vi "LoopScript_ChangeTime.vi"() -> ()   [LabVIEW 2017]
uses:
  FrontPanelReferences.vi
  Desktop/AODExperimentControls/ImageAcquisitionProgram/ImageAcquisitionLibrary/GlobalFrontPanelReferences.vi
  Desktop/AODExperimentControls/AODControl/AODGlobals.vi
  Desktop/AODExperimentControls/AODControl/MessageQueue/QueueOperations/Enqueue Message (Single).vi
  Desktop/AODExperimentControls/ImageAcquisitionProgram/ImageAcquisitionLibrary/ImageAcquisitionLibrary.lvlib
  Desktop/AODExperimentControls/AODControl/AODControl.lvlib
  Desktop/AODExperimentControls/AODControl/MessageQueue/MessageQueue.lvlib
panel:
  out "Current Radius":dbl
  in  "R_f":dbl
  in  "R_0":dbl
  in  "Radius Steps":i32=30
  out "Current Step Down":i32
  out "Current Step Up":i32
  out "Current Loop":i32
  in  "NumberOfLoops":i32
  in  "Record Time":u32=15000
  in  "B_f^2":dbl
  in  "B_0^2":dbl
  in  "Steps":i32=30
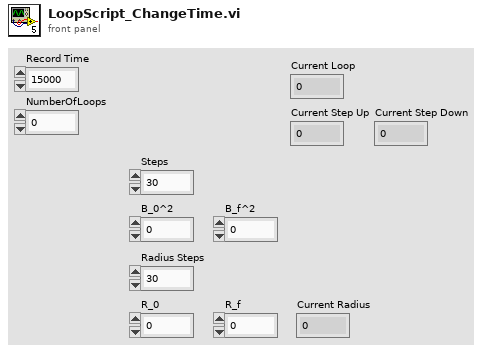
[diagram p1: front panel]
types:
  T1 = typedef "AODControl.lvlib/MessageQueue.lvlib/All Message Queues.ctl" = cluster{" AOD Interface":refnum<queue>}
  T2 = typedef "ImageAcquisitionLibrary.lvlib/References.ctl" = cluster{"Acquire":refnum<vi>, "Rec":refnum<vi>, "Tracking":refnum<vi>, "Settings":refnum<vi>, "Stop":refnum<vi>, "Initialized?":bool, "ImDisplay":refnum<vi>}
  T3 = typedef "WaveformGenerator.lvlib/WaveformGeneratorInterfaceRef.ctl" = cluster{"Waveform X":refnum<vi>, "Waveform Y":refnum<vi>, "Waveform Z":refnum<vi>, "Amplitude X":refnum<vi>, "Amplitude Y":refnum<vi>, "Amplitude Z":refnum<vi>, "Frequency X":refnum<vi>, "Frequency Y":refnum<vi>, "Frequency Z":refnum<vi>, "Phase X":refnum<vi>, "Phase Y":refnum<vi>, "Phase Z":refnum<vi>, "Offset X":refnum<vi>, "Offset Y":refnum<vi>, "Offset Z":refnum<vi>, "Stop":refnum<vi>, "On/Off":refnum<vi>, "Field^2":refnum<vi>}
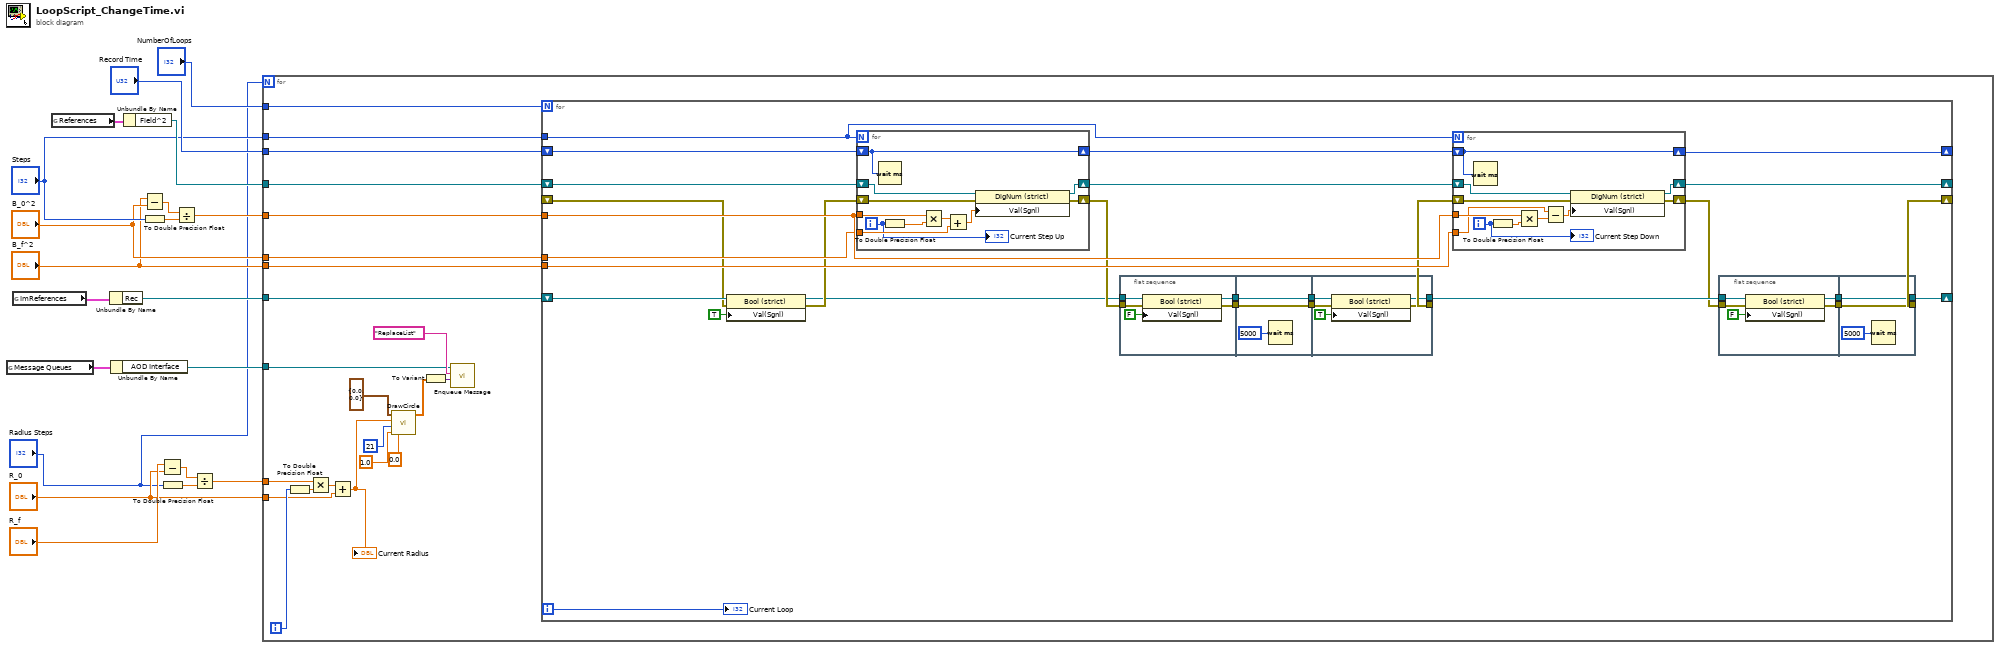
[diagram p0: block diagram]
diagram:
  n1 = global read "AODGlobals.vi" "Message Queues"() -> (w8:T1)
  n2 = global read "GlobalFrontPanelReferences.vi" "ImReferences"() -> (w10:T2)
  n3 = global read "FrontPanelReferences.vi" "References"() -> (w20:T3)
  n4 = Unbundle By Name(w10) -> ("Rec"=w9:refnum<vi>)
  n5 = Unbundle By Name(w8) -> ("AOD Interface"=w7:refnum<queue>)
  n6 = Unbundle By Name(w20) -> ("Field^2"=w19:refnum<vi>)
  n7 = Subtract(x="B_f^2", y="B_0^2") -> (x-y=w17:dbl)
  n8 = To Double Precision Float(number="Steps") -> (double precision float=w18:dbl)
  n9 = Subtract(x="R_f", y="R_0") -> (x-y=w6:dbl)
  n10 = To Double Precision Float(number="Radius Steps") -> (double precision float=w5:dbl)
  n11 = Divide(x=w17, y=w18) -> (x/y=w14:dbl)
  n12 = Divide(x=w6, y=w5) -> (x/y=w3:dbl)
  n13 = for {
    N: "Radius Steps" -> [_]
    tunnel: w19 -> [w42]
    tunnel: "Record Time" -> [w41]
    tunnel: "Steps" -> [w40]
    tunnel: w14 -> [w39]
    tunnel: "B_0^2" -> [w38]
    tunnel: "NumberOfLoops" -> [w37]
    tunnel: "B_f^2" -> [w36]
    tunnel: w9 -> [w35]
    tunnel: w7 -> [w27]
    tunnel: w3 -> [w26]
    tunnel: "R_0" -> [w22]
    i -> [w24]
    n14 = To Double Precision Float(number=w24) -> (double precision float=w25:dbl)
    n15 = Multiply(x=w26, y=w25) -> (x*y=w23:dbl)
    n16 = Add(x=w23, y=w22) -> (x+y=w21:dbl)
    "Current Radius" <- w21
    n17 = call "DrawCircle.vi"("Phase"=0.0, "Eccentricity"=1.0, "No Of Points"=21, "Radius"=w21, "Center"=cluster{"X":dbl, "Y":dbl} {"X"=0.0, "Y"=0.0}) -> ("Array"=w33:dbl[][])  [unwired: 6 in]
    n18 = To Variant(anything=w33) -> (Variant=w34:variant)
    n19 = call-poly "Enqueue Message.vi"("Message Data"=w34, "Message"="ReplaceList", "Message Queue"=w27) -> ()  [unwired: 7 in, 2 out]
    n20 = for {
      N: w37 -> [_]
      tunnel: w40 -> [w68]
      tunnel: w39 -> [w65]
      tunnel: w38 -> [w64]
      shift-right: [w43] -> _
      shift-left: _ -> [w47]
      shift-right: [w61] -> _
      shift-left: w42 -> [w70]
      shift-right: [w62] -> _
      shift-left: w41 -> [w69]
      tunnel: w36 -> [w60]
      shift-right: [w45] -> _
      shift-left: w35 -> [w48]
      i -> [w63]
      n21 = property class="Bool (strict)"(reference=w48, error in=w47, "Val(Sgnl)"=TRUE ("Value (Signaling)")) -> (reference out=w50:refnum<vi>, error out=w51:errorcluster)
      n22 = for {
        N: w68 -> [_]
        shift-right: [w106] -> w66
        shift-left: w70 -> [w113]
        shift-right: [w105] -> w59
        shift-left: w51 -> [w112]
        tunnel: w64 -> [w111]
        tunnel: w65 -> [w109]
        shift-right: [w104] -> w67
        shift-left: w69 -> [w104]
        i -> [w103]
        n23 = Wait (ms)(milliseconds to wait=w104) -> ()  [unwired: 1 out]
        n24 = To Double Precision Float(number=w103) -> (double precision float=w110:dbl)
        n25 = Multiply(x=w109, y=w110) -> (x*y=w108:dbl)
        n26 = Add(x=w108, y=w111) -> (x+y=w107:dbl)
        n27 = property class="DigNum (strict)"(reference=w113, error in=w112, "Val(Sgnl)"=w107) -> (reference out=w106:refnum<vi>, error out=w105:errorcluster)
        "Current Step Up" <- w103
      }
      n28 = flat-sequence {
        tunnel: w59 -> [w83]
        tunnel: w50 -> [w82]
        tunnel: [w80] -> w57
        tunnel: [w79] -> w55
        tunnel: [w85] -> w58
        tunnel: w57 -> [w85]
        tunnel: [w84] -> w56
        tunnel: w55 -> [w84]
        tunnel: w58 -> [w91]
        tunnel: w56 -> [w90]
        tunnel: [w88] -> w46
        tunnel: [w87] -> w54
        frame #0 {
          n29 = property class="Bool (strict)"(reference=w82, error in=w83, "Val(Sgnl)"=FALSE ("Value (Signaling)")) -> (reference out=w80:refnum<vi>, error out=w79:errorcluster)
        }
        frame #1 {
          n30 = Wait (ms)(milliseconds to wait=u32 5000) -> ()  [unwired: 1 out]
        }
        frame #2 {
          n31 = property class="Bool (strict)"(reference=w91, error in=w90, "Val(Sgnl)"=TRUE ("Value (Signaling)")) -> (reference out=w88:refnum<vi>, error out=w87:errorcluster)
        }
      }
      n32 = for {
        N: w68 -> [_]
        shift-right: [w98] -> w61
        shift-left: w66 -> [w102]
        shift-right: [w97] -> w44
        shift-left: w54 -> [w101]
        tunnel: w60 -> [w92]
        tunnel: w65 -> [w99]
        shift-right: [w96] -> w62
        shift-left: w67 -> [w96]
        i -> [w94]
        n33 = Wait (ms)(milliseconds to wait=w96) -> ()  [unwired: 1 out]
        n34 = To Double Precision Float(number=w94) -> (double precision float=w100:dbl)
        n35 = Multiply(x=w99, y=w100) -> (x*y=w93:dbl)
        n36 = Subtract(x=w92, y=w93) -> (x-y=w95:dbl)
        n37 = property class="DigNum (strict)"(reference=w102, error in=w101, "Val(Sgnl)"=w95) -> (reference out=w98:refnum<vi>, error out=w97:errorcluster)
        "Current Step Down" <- w94
      }
      n38 = flat-sequence {
        tunnel: w44 -> [w75]
        tunnel: w46 -> [w74]
        tunnel: [w72] -> w53
        tunnel: [w71] -> w52
        tunnel: w53 -> [w77]
        tunnel: w52 -> [w76]
        tunnel: [w77] -> w45
        tunnel: [w76] -> w43
        frame #0 {
          n39 = property class="Bool (strict)"(reference=w74, error in=w75, "Val(Sgnl)"=FALSE ("Value (Signaling)")) -> (reference out=w72:refnum<vi>, error out=w71:errorcluster)
        }
        frame #1 {
          n40 = Wait (ms)(milliseconds to wait=u32 5000) -> ()  [unwired: 1 out]
        }
      }
      "Current Loop" <- w63
    }
  }
